vi "Filter Get Averaging Factor.vi"(11 "averagingFactor":i32) -> (2 "function return":u32, 3 "averagingFactor out":i32)   [LabVIEW 2018, in "Copy of Andor SDK.lvlib"]
doc: "EXPNETTYPE unsigned int WINAPI Filter_GetAveragingFactor(int * averagingFactor);"
uses:
  Copy of Andor SDK.lvlib
  <userlib>/Andor SDK/ATMCD32D.dll
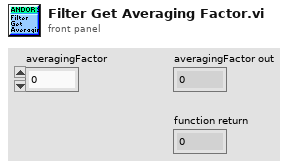
[diagram p1: front panel]
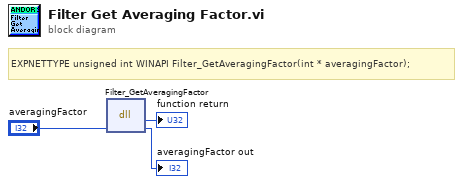
[diagram p0: block diagram]
diagram:
  # "EXPNETTYPE unsigned int WINAPI Filter_GetAveragingFactor(int * averagingFactor);"
  n1 = dll-call lib="C:/Program Files (x86)/National Instruments/LabVIEW 2018/user.lib/Andor SDK/ATMCD32D.*" fn="Filter_GetAveragingFactor"("averagingFactor"="averagingFactor") -> (→"function return":u32, "averagingFactor"=→"averagingFactor out":i32)  [unwired: 3 in, 2 out]
